vi "test harness_FXP_Matrix_Vector_mult_loop_32bit.vi"(8 "error in (no error)":errorcluster, 11 "TestCase in":refnum<class "FXP_observer_TestCase.lvclass">) -> (0 "error out":errorcluster, 3 "TestCase out":refnum<class "FXP_observer_TestCase.lvclass">)   [LabVIEW 2019, in "FXP_observer_TestCase.lvclass"]
uses:
  FXP_observer_TestCase.lvclass
  C:/Program Files (x86)/National Instruments/LabVIEW 2019/vi.lib/addons/_JKI Toolkits/VI Tester/TestCase.llb/TestCase.lvclass
  <vilib>/rvi/DesktopExecutionNode/Execution/niFpgaDEN_Execute.vi
  <vilib>/rvi/DesktopExecutionNode/DesktopExecutionNode.xnode
  <vilib>/Wiresmith Technology/VITAC (VI Tester Advanced Comparisons)/VITAC.lvlib
panel:
  out "size(s)":i32
  out "error out 2":errorcluster
  out "xk_1_1_mem":fxp<+/-,32,5>[](array[numeric])
  out "xk_0_1 (mem)":fxp<+/-,32,7>[](array[numeric])
  out "A*xk (expected)":fxp<+/-,64,12>[](array[numeric])
  in  "Az_mat":fxp<+/-,32,5>[][](array[numeric])=[[1.0, 2.0, 3.0, 4.0], [1.0, 2.0, 2.0, 3.0], [-4.0, -1.0, -3.0, -2.0], [1.0, 5.0, 1.0, 2.0]]
  in  "x_k":fxp<+/-,32,5>[](array[numeric])=[0.10000000149011612, 0.20000000298023224, 0.29999999701976776, 0.3999999985098839, 0.0, 0.0, 0.0, 0.0, 0.0, 0.0, 0.0, 0.0, 0.0, 0.0, 0.0, 0.0, 0.0, 0.0, 0.0, 0.0, 0.0, 0.0, 0.0, 0.0, 0.0, 0.0, 0.0, 0.0, 0.0, 0.0, 0.0, 0.0, 0.0, 0.0, 0.0, 0.0, 0.0, 0.0, 0.0, 0.0, 0.0, 0.0, 0.0, 0.0, 0.0, 0.0, 0.0, 0.0, 0.0, 0.0]
  in  "NS":u8=4
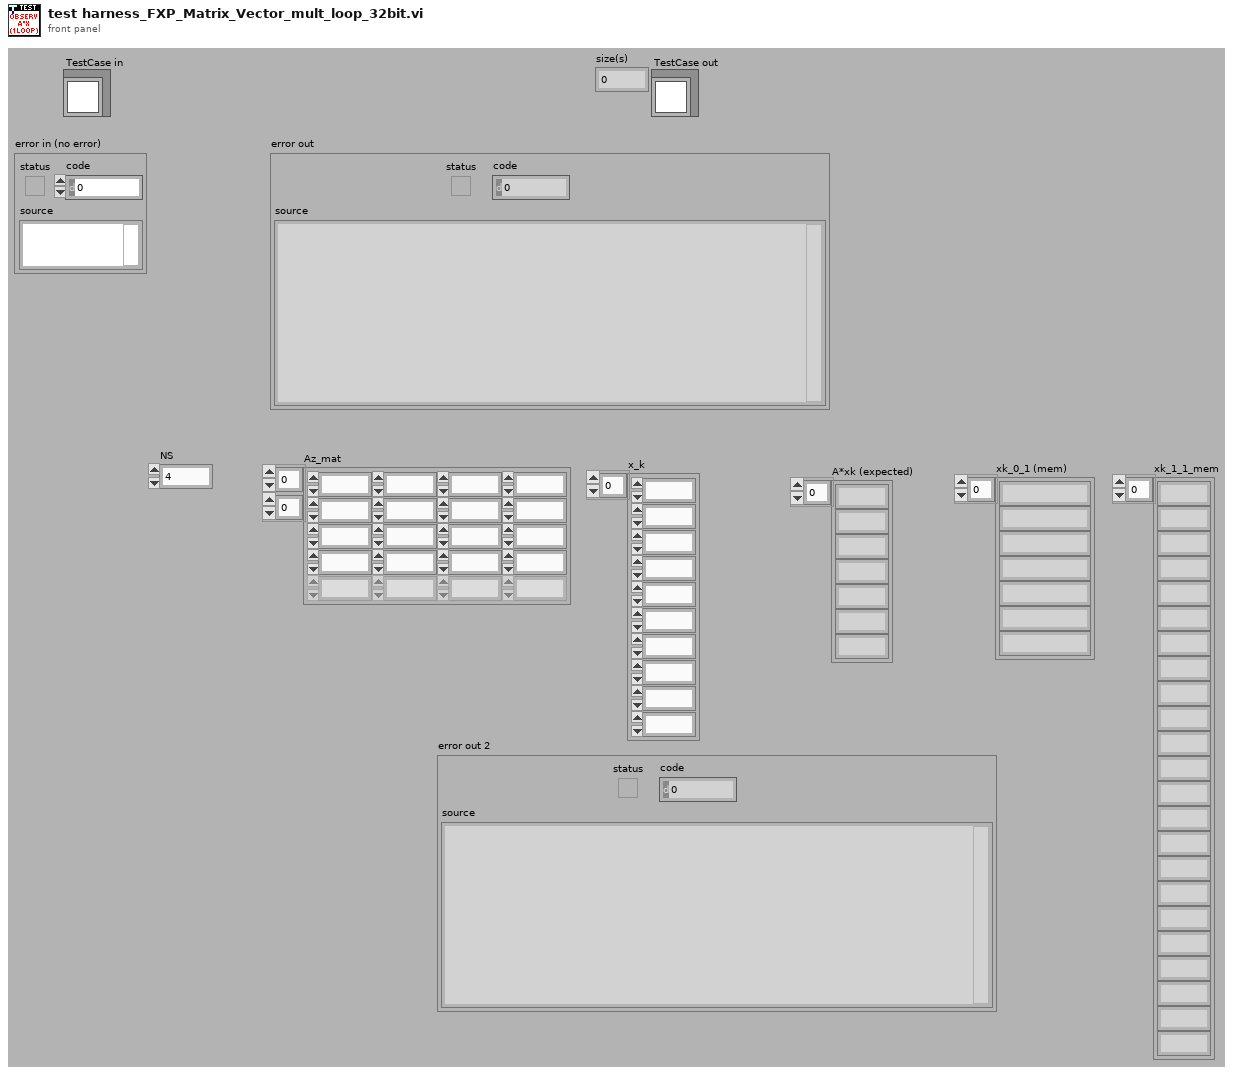
[diagram p1: front panel]
types:
  T1 = typedef "x_vec_type.ctl" = fxp<+/-,32,6>[]
  T2 = typedef "Az_vec_scalar.ctl" = fxp<+/-,32,7>
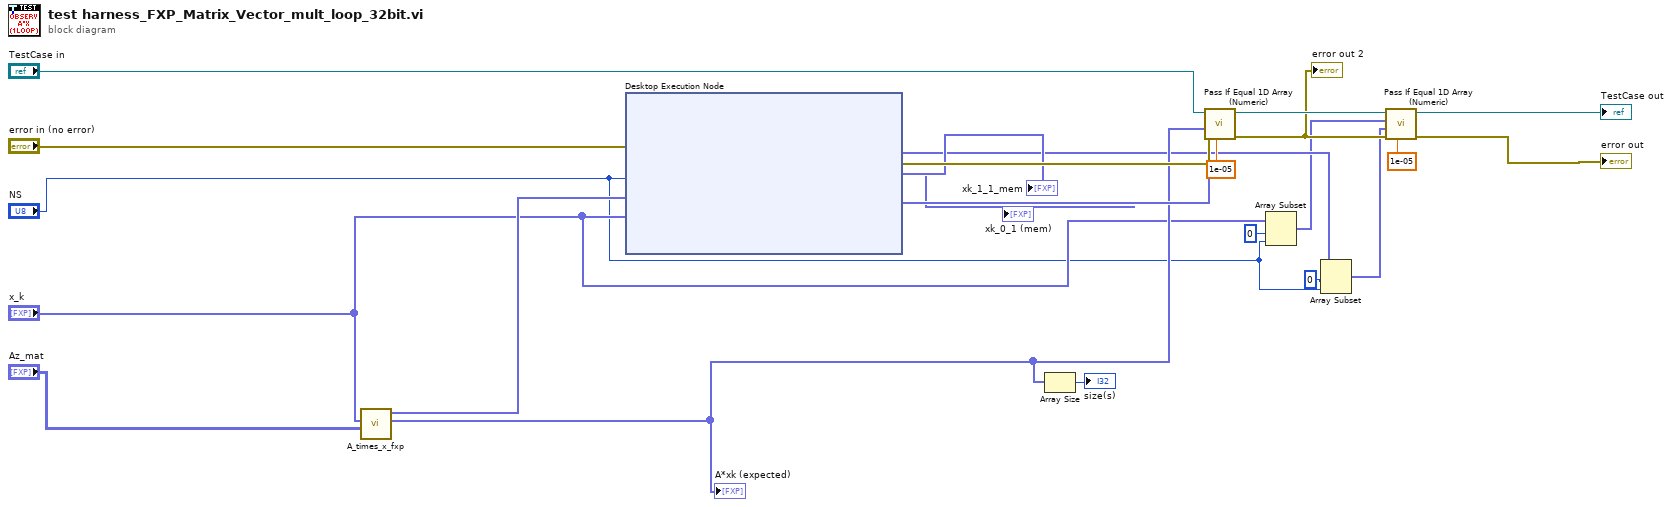
[diagram p0: block diagram]
diagram:
  n1 = call "A_times_x_fxp.vi"("Az_mat in"="Az_mat", "x_vec"="x_k") -> ("A*x"=w9:T1, "Az_vec out"=w19:T2[])  [unwired: 8 in]
  "A*xk (expected)" <- w9
  n2 = xnode "Desktop Execution Node"("Error In"="error in (no error)", "NS"="NS", "Az_col"=w19, "x_k"="x_k") -> ("Error Out"=w16:errorcluster, "Ax (xk_1_0)"=w15:fxp<+/-,32,6>[], "xk_0_1"=w6:fxp<+/-,32,6>[])
  "xk_0_1 (mem)" <- w6
  "xk_1_1_mem" <- w15
  n3 = Array Size(array=w9) -> (size(s)=→"size(s)":i32)
  n4 = call <vilib>:"Pass If Equal 1D Array (Numeric).vi"("delta (optional)"=1e-05 ("del u_x"), "error in (no error)"=w16, "actual"=w9, "expected"=w15, "TestCase in"="TestCase in") -> ("error out"=w10:errorcluster, "TestCase out"=w12:refnum<class "FXP_observer_TestCase.lvclass">)  [unwired: 5 in]
  "error out 2" <- w10
  n5 = Array Subset(array="x_k", index=0, length="NS") -> (w4:fxp<+/-,32,5>[])
  n6 = Array Subset(array=w6, index=0, length="NS") -> (w5:fxp<+/-,32,6>[])
  n7 = call <vilib>:"Pass If Equal 1D Array (Numeric).vi"("delta (optional)"=1e-05 ("del u_x"), "error in (no error)"=w10, "actual"=w5, "expected"=w4, "TestCase in"=w12) -> ("error out"=→"error out":errorcluster, "TestCase out"=→"TestCase out":refnum<class "FXP_observer_TestCase.lvclass">)  [unwired: 5 in]
